vi "meanAngle.vi"(1 "steering_is":T1) -> (0 "Numeric":dbl)   [LabVIEW 2016]
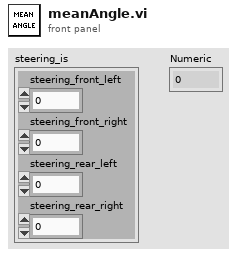
[diagram p1: front panel]
types:
  T1 = cluster{"steering_front_left":dbl, "steering_front_right":dbl, "steering_rear_left":dbl, "steering_rear_right":dbl}
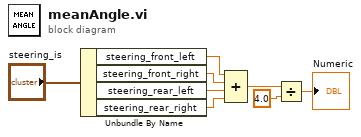
[diagram p0: block diagram]
diagram:
  n1 = Unbundle By Name("steering_is") -> ("steering_front_left"=w2:dbl, "steering_front_right"=w3:dbl, "steering_rear_left"=w4:dbl, "steering_rear_right"=w5:dbl)
  n2 = Compound Arithmetic op=ADD(w2, w3, w4, w5) -> (w6:dbl)
  n3 = Divide(x=w6, y=4.0) -> (x/y=→"Numeric":dbl)
